vi "RefToData.vi"(8 "error in (no error)":errorcluster, 11 ".NET Refnum in":refnum<k24>) -> (0 "error out":errorcluster, 3 "variant out":variant)   [LabVIEW 2020, in "ORM_Dapper.lvlib" / "DapperRow.lvclass"]
uses:
  DapperRow.lvclass
  DapperRow.lvclass/DapperRow.ctl
panel:
  out "Array":string[][](array[string])
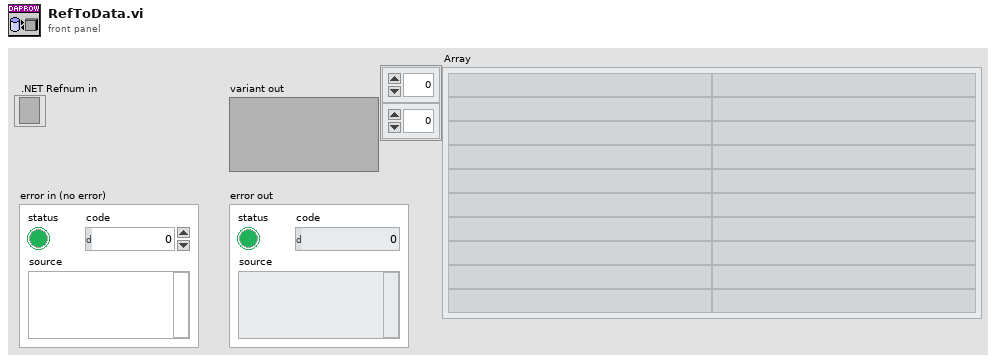
[diagram p1: front panel]
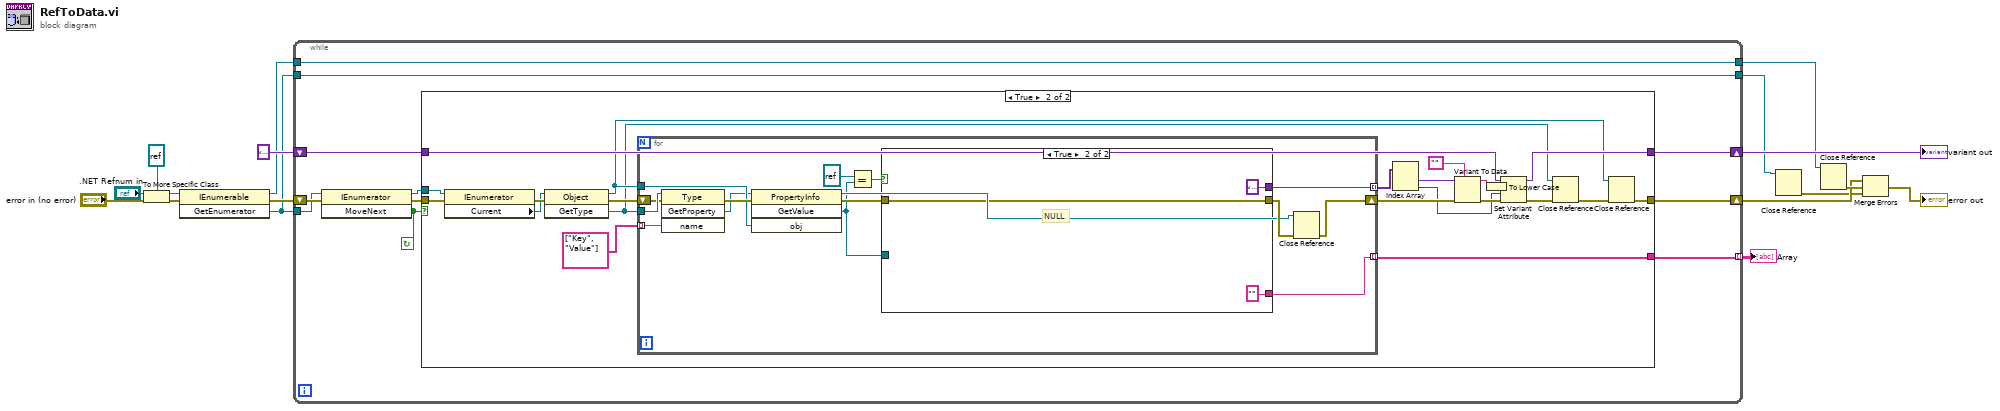
[diagram p0: block diagram]
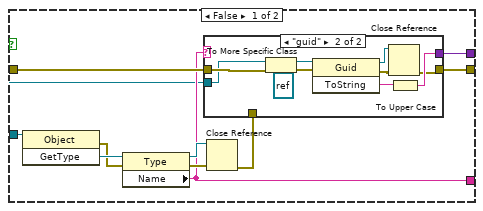
[diagram p3: hidden frame]
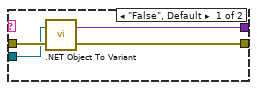
[diagram p4: hidden frame]
diagram:
  n1 = To More Specific Class(target class=refnum<k24> refnum ("reference"), reference=".NET Refnum in", error in="error in (no error)") -> (specific class reference=w11:refnum<k24>, error out=w13:errorcluster)
  n2 = invoke class="IEnumerable" method="GetEnumerator"(reference=w11, error in=w13) -> (reference out=w9:refnum<k24>, error out=w15:errorcluster, "GetEnumerator"=w3:refnum<k24>)  [unwired: 1 in]
  n3 = while {
    tunnel: w3 -> [w21]
    shift-right: [w25] -> w16
    shift-left: variant ("variant out") -> [w26]
    shift-right: [w22] -> w6
    shift-left: w15 -> [w24]
    tunnel: w9 -> [w20]
    tunnel: [w20] -> w5
    tunnel: w3 -> [w19]
    tunnel: [w19] -> w2
    tunnel: [w18] -> w1 mode=indexing
    stop <- w27 continue-if-true
    n4 = invoke class="IEnumerator" method="MoveNext"(reference=w21, error in=w24) -> (reference out=w28:refnum<k24>, error out=w23:errorcluster, "MoveNext"=w27:bool)  [unwired: 1 in]
    n5 = case shown="True" w27 {
      tunnel: w28 -> [_ w40]
      tunnel: w26 -> [w30 w50]
      tunnel: [w30 w41] -> w25
      tunnel: w23 -> [w29 w46]
      tunnel: [w29 w36] -> w22
      tunnel: [_ w31] -> w18
      frame False {
      }
      frame True {
        n6 = property class="IEnumerator"(reference=w40, error in=w46) -> (error out=w45:errorcluster, "Current"=w37:refnum<k24>)  [unwired: 1 out]
        n7 = invoke class="Object" method="GetType"(reference=w37, error in=w45) -> (reference out=w35:refnum<k24>, error out=w44:errorcluster, "GetType"=w33:refnum<k24>)  [unwired: 1 in]
        n8 = for {
          tunnel: w33 -> [w67]
          tunnel: string[] ["Key", "Value"] ("Array 2") -> [w66] mode=indexing
          tunnel: w35 -> [w61]
          tunnel: [w65] -> w51 mode=indexing
          shift-right: [w59] -> w39
          shift-left: w44 -> [w64]
          tunnel: [w56] -> w31 mode=indexing
          n9 = invoke class="Type" method="GetProperty"(reference=w67, error in=w64, "name"=w66) -> (error out=w63:errorcluster, "GetProperty"=w57:refnum<k24>)  [unwired: 1 in, 2 out]
          n10 = invoke class="PropertyInfo" method="GetValue"(reference=w57, error in=w63, "obj"=w61) -> (reference out=w58:refnum<k24>, error out=w62:errorcluster, "GetValue"=w55:refnum<k24>)  [unwired: 1 in, 1 out]
          n11 = Equal?(x=refnum<k24> refnum, y=w55) -> (x = y?=w53:bool)
          n12 = case shown="True" w53 {
            tunnel: [w77 variant ("variant")] -> w65
            tunnel: w62 -> [w76 w94]
            tunnel: [w75 w94] -> w60
            tunnel: [w71 "" ("Name")] -> w56
            tunnel: w55 -> [w68 _]
            frame False {
              n13 = invoke class="Object" method="GetType"(reference=w68) -> (error out=w69:errorcluster, "GetType"=w74:refnum<k24>)  [unwired: 2 in, 1 out]
              n14 = property class="Type"(reference=w74, error in=w69) -> (reference out=w72:refnum<k24>, error out=w73:errorcluster, "Name"=w71:string)
              n15 = Close Reference(reference=w72, error in (no error)=w73) -> (error out=w70:errorcluster)
              n16 = case shown="\"guid\"" w71 {
                tunnel: [w81 w85] -> w77
                tunnel: w76 -> [w80 w87]
                tunnel: [w79 w82] -> w75
                tunnel: w68 -> [w78 w86]
                tunnel: w70 -> [_ _]
                frame "False", Default {
                  n17 = call <vilib>:".NET Object To Variant.vi"("error in (no error)"=w80, ".NET object"=w78) -> ("error out"=w79:errorcluster, "variant"=w81:variant)
                }
                frame "guid" {
                  n18 = To More Specific Class(target class=refnum<k24> refnum ("NewGuid"), reference=w86, error in=w87) -> (specific class reference=w90:refnum<k24>, error out=w89:errorcluster)
                  n19 = invoke class="Guid" method="ToString"(reference=w90, error in=w89) -> (reference out=w83:refnum<k24>, error out=w84:errorcluster, "ToString"=w91:string)  [unwired: 1 in]
                  n20 = Close Reference(reference=w83, error in (no error)=w84) -> (error out=w82:errorcluster)
                  n21 = To Upper Case(1:w91) -> (0:w85:string)
                }
              }
            }
            frame True {
              # "NULL"
            }
          }
          n22 = Close Reference(reference=w58, error in (no error)=w60) -> (error out=w59:errorcluster)
        }
        n23 = Index Array(array=w51) -> (element #1=w49:variant, element #2=w38:variant)  [unwired: 2 in]
        n24 = Variant To Data(error in=w39, type="", Variant=w49) -> (data=w47:string, error out=w43:errorcluster)
        n25 = To Lower Case(string=w47) -> (all lower case string=w32:string)
        n26 = Set Variant Attribute(Variant=w50, name=w32, value=w38, error in=w43) -> (Variant out=w41:variant, error out=w42:errorcluster)  [unwired: 1 out]
        n27 = Close Reference(reference=w33, error in (no error)=w42) -> (error out=w34:errorcluster)
        n28 = Close Reference(reference=w35, error in (no error)=w34) -> (error out=w36:errorcluster)
      }
    }
  }
  "variant out" <- w16
  "Array" <- w1
  n29 = Close Reference(reference=w2) -> (error out=w4:errorcluster)  [unwired: 1 in]
  n30 = Close Reference(reference=w5) -> (error out=w8:errorcluster)  [unwired: 1 in]
  n31 = Merge Errors(w6, w8, w4) -> (→"error out":errorcluster)
